vi "Focus_Ctrl_Index.vi"(8 "NewVal":variant, 9 "OldVal":variant) -> (2 "Focus out":T1, 3 "Control out":refnum<vi>)   [LabVIEW 2011]
uses:
  Controls/Focus.ctl
panel:
  in  "Focus in":T1
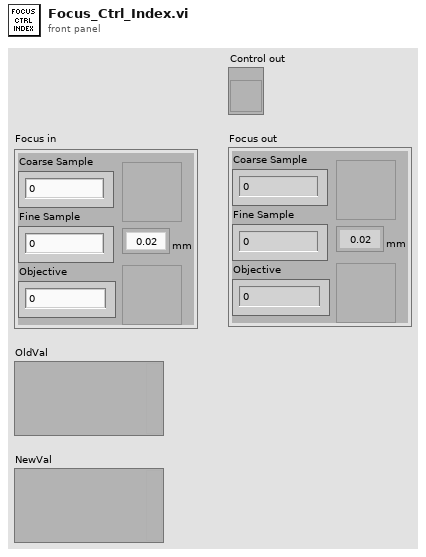
[diagram p1: front panel]
types:
  T1 = typedef "Focus.ctl" = cluster{"Focus Step (um)":enum16{"0.02", "0.05", "0.1", "0.5", "1", "2", "5", "10", "20"}, "Focus Up":bool, "Focus Down":bool, "M227":dbl, "P541":dbl, "N664":dbl}
  T2 = cluster{"Focus Step (um)":bool, "Focus Up":bool, "Focus Down":bool, "M227":bool, "P541":bool, "N664":bool}
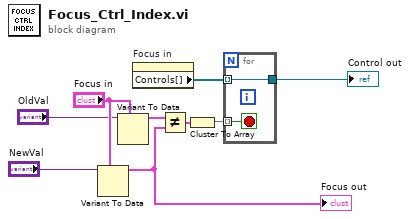
[diagram p0: block diagram]
diagram:
  n1 = Variant To Data(type="Focus in", Variant="NewVal") -> (data=w9:T1)  [unwired: 1 in, 1 out]
  "Focus out" <- w9
  n2 = Variant To Data(type="Focus in", Variant="OldVal") -> (data=w3:T1)  [unwired: 1 in, 1 out]
  n3 = property on="Focus in" class="Clust"() -> ("Controls[]"=w1:refnum<vi>[])  [unwired: 2 in, 2 out]
  n4 = Not Equal?(x=w3, y=w9) -> (x != y?=w7:T2)
  n5 = Cluster To Array(cluster=w7) -> (array=w4:bool[])
  n6 = for {
    tunnel: w4 -> [w10] mode=indexing
    tunnel: w1 -> [w11] mode=indexing
    tunnel: [w11] -> w2
    stop <- w10 stop-if-true
  }
  "Control out" <- w2
